vi "uc480_SubVI_Example_Timing.vi"(0 ".NET (Reference)":refnum<k24>, 5 "Pixelclock":i32, 7 "Exposure time":dbl, 9 "Framerate":dbl, 11 "Error In":errorcluster) -> (6 "Pixelclock":i32, 8 "Exposure time":dbl, 10 "Framerate":dbl, 15 "Error Out":errorcluster)   [LabVIEW 2016]
uses:
  C:/Users/Anatec i3/Desktop/Labview Projects/IR OPO Controller/Branches/XPS version/uc480DotNet.dll
  uc480DotNet.dll
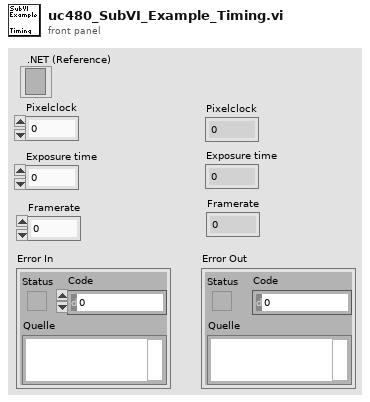
[diagram p1: front panel]
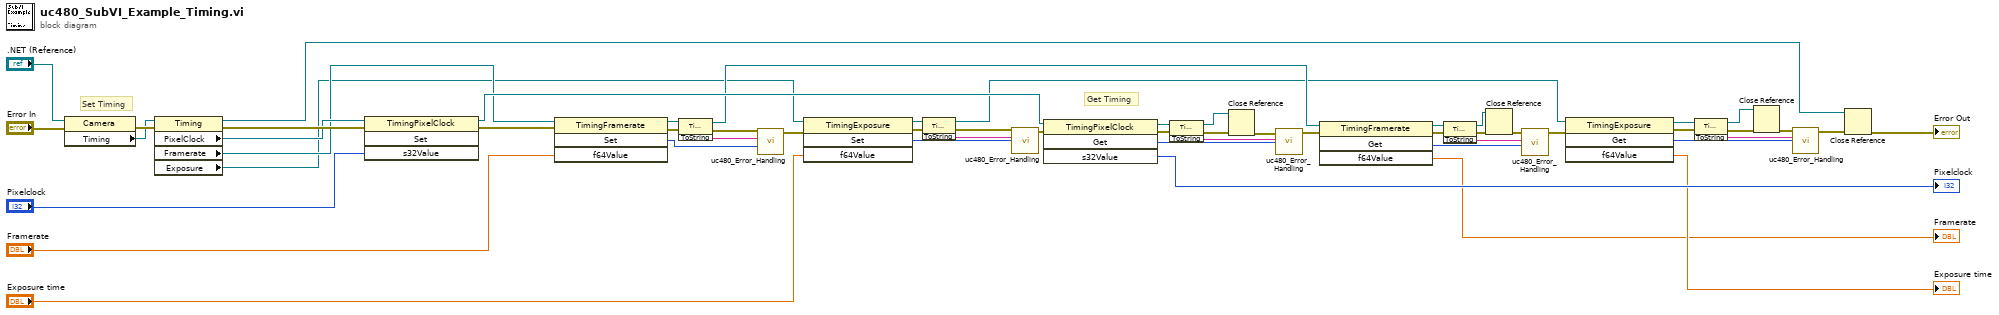
[diagram p0: block diagram]
diagram:
  # "Get Timing"
  # "Set Timing"
  n1 = property class="Camera"(reference=".NET (Reference)", error in="Error In") -> (error out=w43:errorcluster, "Timing"=w42:refnum<k24>)  [unwired: 1 out]
  n2 = property class="Timing"(reference=w42, error in=w43) -> (reference out=w7:refnum<k24>, error out=w13:errorcluster, "PixelClock"=w6:refnum<k24>, "Framerate"=w4:refnum<k24>, "Exposure"=w2:refnum<k24>)
  n3 = invoke class="TimingPixelClock" method="Set"(reference=w6, error in=w13, "s32Value"="Pixelclock") -> (reference out=w5:refnum<k24>, error out=w12:errorcluster)  [unwired: 1 in, 2 out]
  n4 = invoke on="Methodenknoten" class="TimingFramerate" method="Set"(reference=w4, error in=w12, "f64Value"="Framerate") -> (reference out=w55:refnum<k24>, error out=w54:errorcluster, "Set"=w53:i32)  [unwired: 1 in, 1 out]
  n5 = invoke class="TimingFramerate" method="ToString"(reference=w55, error in=w54) -> (reference out=w3:refnum<k24>, error out=w11:errorcluster, "ToString"=w52:string)  [unwired: 1 in]
  n6 = call "uc480_Error_Handling.vi"("Error Code"=w53, "Error String"=w52, "Error In"=w11) -> ("Error Out"=w56:errorcluster)  [unwired: 8 in]
  n7 = invoke class="TimingExposure" method="Set"(reference=w2, error in=w56, "f64Value"="Exposure time") -> (reference out=w46:refnum<k24>, error out=w47:errorcluster, "Set"=w48:i32)  [unwired: 1 in, 1 out]
  n8 = invoke class="TimingExposure" method="ToString"(reference=w46, error in=w47) -> (reference out=w1:refnum<k24>, error out=w10:errorcluster, "ToString"=w49:string)  [unwired: 1 in]
  n9 = call "uc480_Error_Handling.vi"("Error Code"=w48, "Error String"=w49, "Error In"=w10) -> ("Error Out"=w35:errorcluster)  [unwired: 8 in]
  n10 = invoke class="TimingPixelClock" method="Get"(reference=w5, error in=w35) -> (reference out=w39:refnum<k24>, error out=w38:errorcluster, "Get"=w36:i32, "s32Value"=→"Pixelclock":i32)  [unwired: 2 in]
  n11 = invoke class="TimingPixelClock" method="ToString"(reference=w39, error in=w38) -> (reference out=w14:refnum<k24>, error out=w16:errorcluster, "ToString"=w37:string)  [unwired: 1 in]
  n12 = Close Reference(reference=w14, error in (no error)=w16) -> (error out=w15:errorcluster)
  n13 = call "uc480_Error_Handling.vi"("Error Code"=w36, "Error String"=w37, "Error In"=w15) -> ("Error Out"=w26:errorcluster)  [unwired: 8 in]
  n14 = invoke class="TimingFramerate" method="Get"(reference=w3, error in=w26) -> (reference out=w34:refnum<k24>, error out=w33:errorcluster, "Get"=w31:i32, "f64Value"=→"Framerate":dbl)  [unwired: 2 in]
  n15 = invoke class="TimingFramerate" method="ToString"(reference=w34, error in=w33) -> (reference out=w17:refnum<k24>, error out=w19:errorcluster, "ToString"=w32:string)  [unwired: 1 in]
  n16 = Close Reference(reference=w17, error in (no error)=w19) -> (error out=w18:errorcluster)
  n17 = call "uc480_Error_Handling.vi"("Error Code"=w31, "Error String"=w32, "Error In"=w18) -> ("Error Out"=w25:errorcluster)  [unwired: 8 in]
  n18 = invoke class="TimingExposure" method="Get"(reference=w1, error in=w25) -> (reference out=w30:refnum<k24>, error out=w29:errorcluster, "Get"=w27:i32, "f64Value"=→"Exposure time":dbl)  [unwired: 2 in]
  n19 = invoke class="TimingExposure" method="ToString"(reference=w30, error in=w29) -> (reference out=w22:refnum<k24>, error out=w21:errorcluster, "ToString"=w28:string)  [unwired: 1 in]
  n20 = Close Reference(reference=w22, error in (no error)=w21) -> (error out=w20:errorcluster)
  n21 = call "uc480_Error_Handling.vi"("Error Code"=w27, "Error String"=w28, "Error In"=w20) -> ("Error Out"=w9:errorcluster)  [unwired: 8 in]
  n22 = Close Reference(reference=w7, error in (no error)=w9) -> (error out=→"Error Out":errorcluster)
